vi "Unlock VI.vi"(1 "VI File":path) -> (0 "no Error":bool)   [LabVIEW 2020, in "LeMaal.lvlib"]
uses:
  LeMaal.lvlib
  clFile/clFile.lvclass
  clLabview/clLabview.lvclass
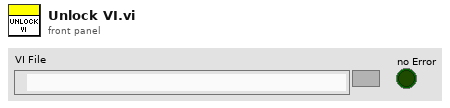
[diagram p1: front panel]
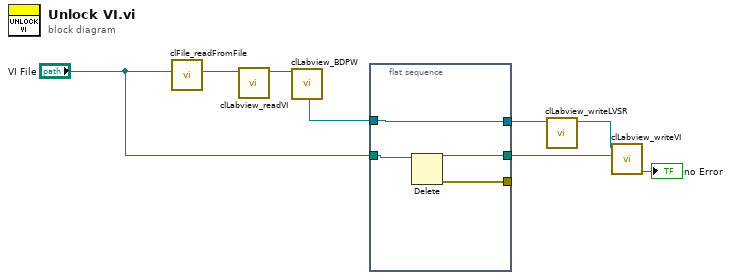
[diagram p0: block diagram]
diagram:
  n1 = call "clFile_readFromFile.vi"("file (use dialog)"="VI File") -> ("clFileReader.lvclass"=w8:refnum<class "clFileReader.lvclass">)  [unwired: 1 in, 9 out]
  n2 = call "clLabview_readVI.vi"("vi_lib.lvlib:clFileReader.lvclass"=w8) -> ("vi_lib.lvlib:clLabview.lvclass 2"=w7:refnum<class "clLabview.lvclass">)  [unwired: 10 out]
  n3 = call "clLabview_BDPW.vi"("vi_lib.lvlib:clLabview.lvclass"=w7) -> ("vi_lib.lvlib:clLabview.lvclass [Out]"=w3:refnum<class "clLabview.lvclass">)  [unwired: 18 out]
  n4 = flat-sequence {
    tunnel: "VI File" -> [w12]
    tunnel: [w11] -> _
    tunnel: [w10] -> w5
    tunnel: w3 -> [w9]
    tunnel: [w9] -> w2
    frame #0 {
      n5 = Delete(path (use dialog)=w12) -> (deleted path=w10:path, error out=w11:errorcluster)  [unwired: 4 in, 1 out]
    }
  }
  n6 = call "clLabview_writeLVSR.vi"("vi_lib.lvlib:clLabview.lvclass"=w2) -> ("vi_lib.lvlib:clLabview.lvclass [Out]"=w1:refnum<class "clLabview.lvclass">)  [unwired: 9 in]
  n7 = call "clLabview_writeVI.vi"("vi_lib.lvlib:clLabview.lvclass"=w1, "filename (use dialog)"=w5) -> ("no Error"=→"no Error":bool)  [unwired: 1 in, 7 out]
